vi "EOL Set Power Supply Voltage.vi"(4 "PS Channel Control":i32, 6 "station name":string, 7 "power supply type":T1, 8 "Error Table In":string[][](table), 9 "station idx":i32=4, 10 "Power Supply Voltage":dbl, 11 "Power Supply Comm Port":refnum<visa-resource-name>="COM1") -> (0 "Error Table Out":string[][](array[string]), 2 "Actual Voltage":dbl, 3 "Pass?":bool)   [LabVIEW 2018]
uses:
  05.UserVI's/Lambda Power/power supply types.ctl
  Fergus/ZUP_Current/Def Ctrl/CMD Type.ctl
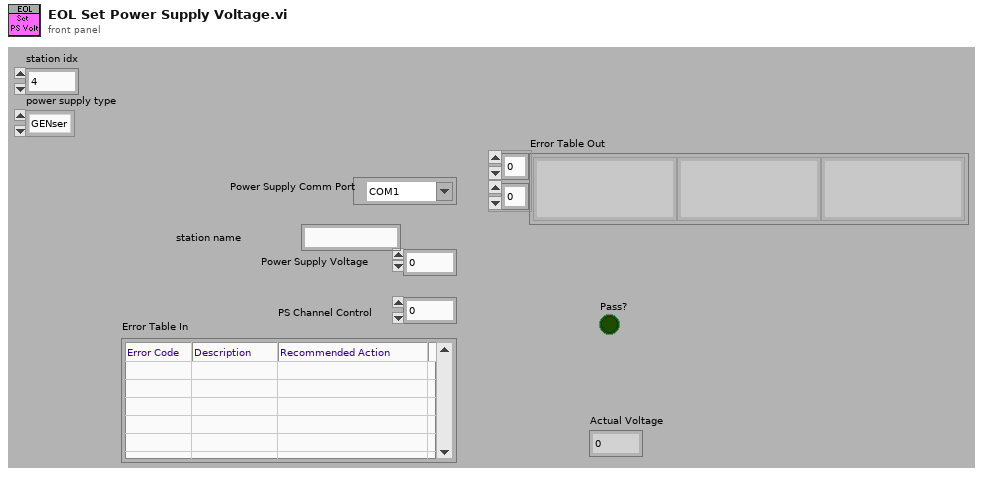
[diagram p1: front panel]
types:
  T1 = typedef "power supply types.ctl" = enum16{"GENser", "ZUPser", "GENeth", "Manual", "ITECH"}
  T2 = cluster{"Power Supply Voltage":dbl, "station name":string, "Max Voltage":dbl, "Min Voltage":dbl, "PS Channel Control":i32, "Power Supply Comm Port":refnum<visa-resource-name>, "Error String":string, "Actual Voltage":dbl, "Start Timer":u32, "Pass?":bool, "station idx":i32, "power supply type":T1}
  T3 = typedef "CMD Type.ctl" = enum16{"Default", "SetADR", "SetRMT", "SetVOL", "SetCUR", "SetOUT", "CheckREV", "CheckRMT", "CheckVOL", "CkeckCUR", "CheckOUT"}
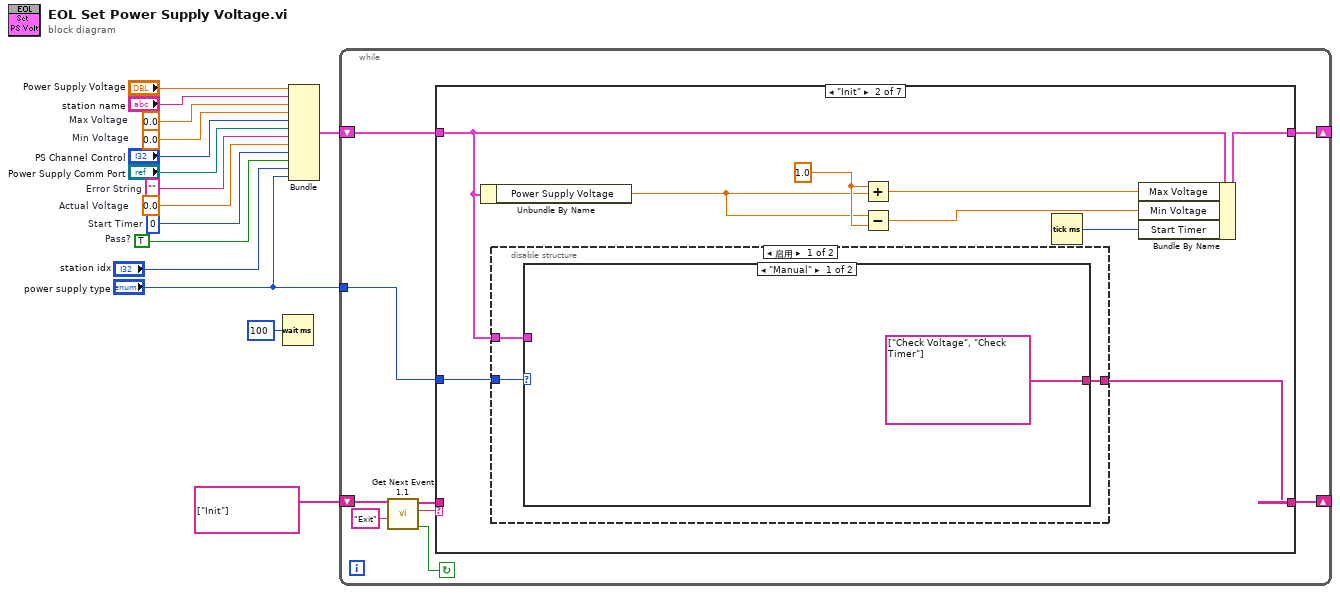
[diagram p0: block diagram]
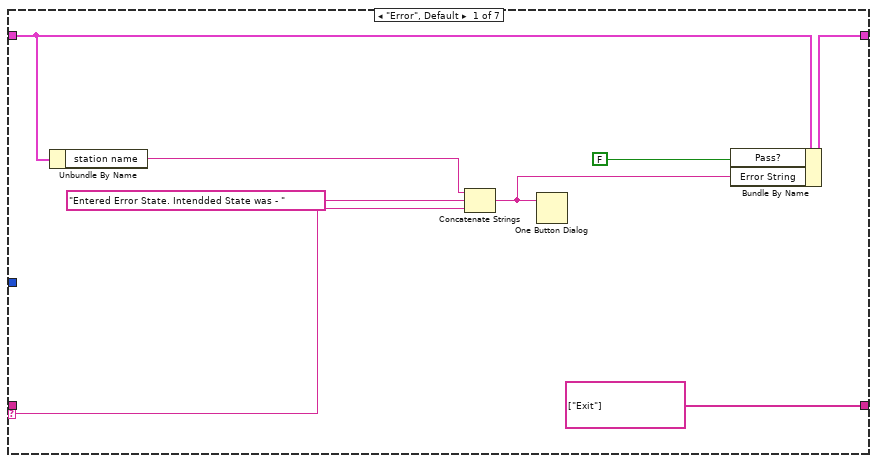
[diagram p2: hidden frame]
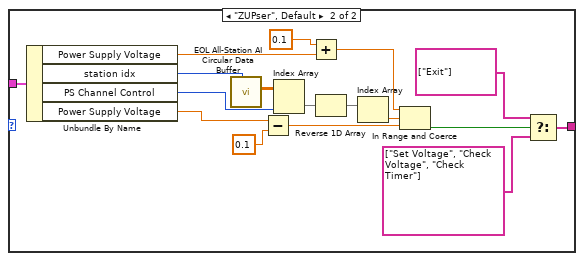
[diagram p3: hidden frame]
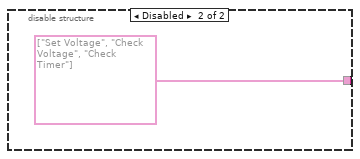
[diagram p4: hidden frame]
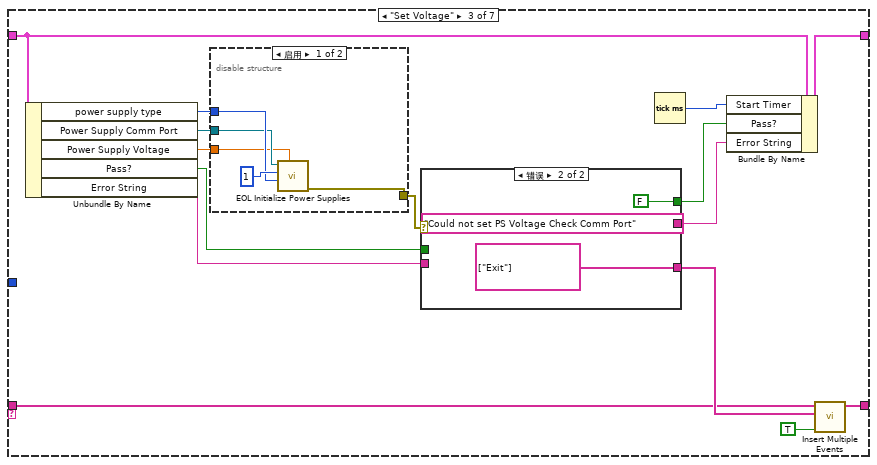
[diagram p5: hidden frame]
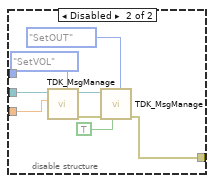
[diagram p6: hidden frame]
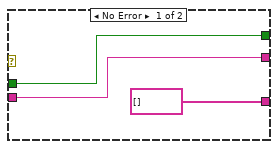
[diagram p7: hidden frame]
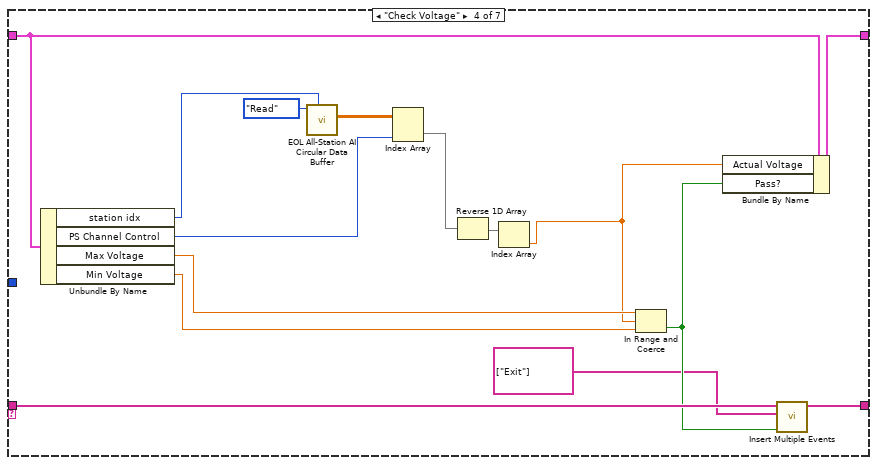
[diagram p8: hidden frame]
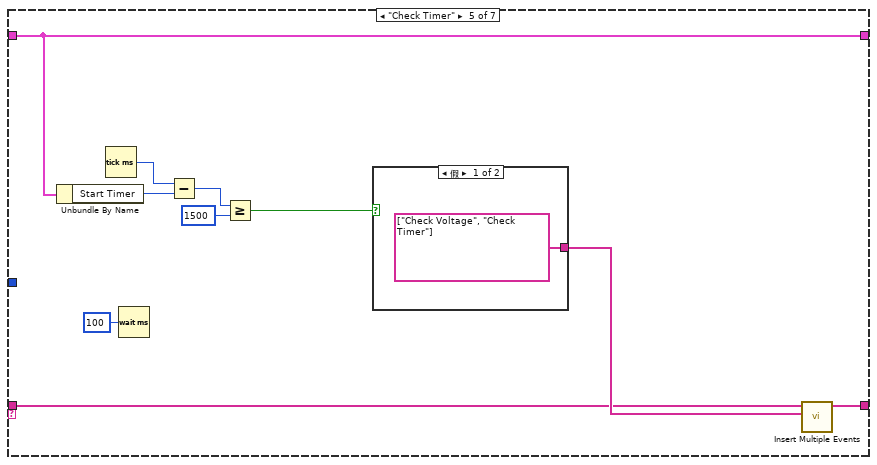
[diagram p9: hidden frame]
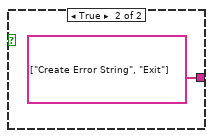
[diagram p10: hidden frame]
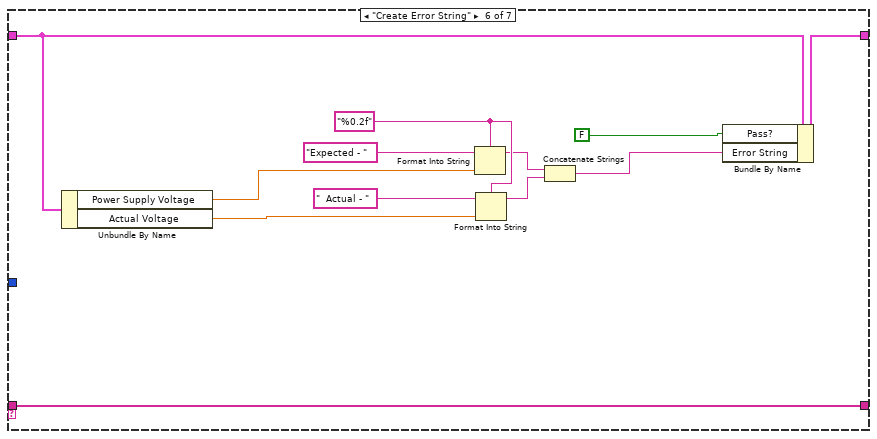
[diagram p11: hidden frame]
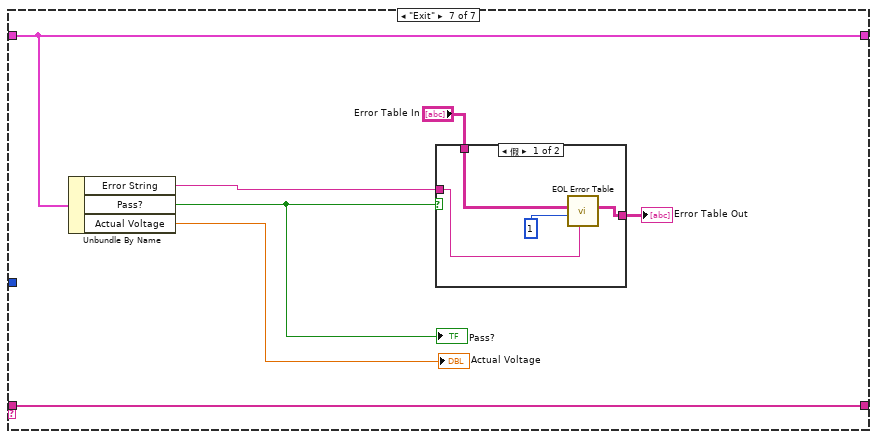
[diagram p12: hidden frame]
diagram:
  w4 = TRUE  # Pass?
  w5 = u32 0  # Start Timer
  w6 = 0.0  # Actual Voltage
  w7 = ""  # Error String
  w11 = 0.0  # Max Voltage
  w10 = 0.0  # Min Voltage
  n1 = Wait (ms)(milliseconds to wait=u32 100) -> ()  [unwired: 1 out]
  n2 = Bundle("Power Supply Voltage"="Power Supply Voltage", "station name"="station name", "Max Voltage"=w11, "Min Voltage"=w10, "PS Channel Control"="PS Channel Control", "Power Supply Comm Port"="Power Supply Comm Port", "Error String"=w7, "Actual Voltage"=w6, "Start Timer"=w5, "Pass?"=w4, "station idx"="station idx", "power supply type"="power supply type") -> (w12:T2)  [unwired: 1 in]
  n3 = while {
    shift-right: [w20] -> _
    shift-left: string[] ["Init"] ("event queue out") -> [w19]
    shift-right: [w17] -> _
    shift-left: w12 -> [w18]
    tunnel: "power supply type" -> [w16]
    stop <- w24 continue-if-true
    n4 = call "Get Next Event 1.1.vi"("Exit Event"="Exit", "event queue in"=w19) -> ("Condition (Exit:F)"=w24:bool, "next event"=w22:string, "event queue out"=w21:string[])  [unwired: 6 in, 1 out]
    n5 = case shown="\"Init\"" w22 {
      selector: w22 -> [w31 _ _ _ _ _ _]
      tunnel: w21 -> [_ _ w76 w106 w115 w136 w143]
      tunnel: [string[] ["Exit"] ("event queue out") w34 w78 w107 w116 w136 w143] -> w20
      tunnel: w18 -> [w29 w35 w74 w109 w114 w135 w140]
      tunnel: [w28 w39 w73 w108 w114 w134 w140] -> w17
      tunnel: w16 -> [_ w33 _ _ _ _ _]
      frame "Error", Default {
        n6 = Unbundle By Name(w29) -> ("station name"=w25:string)
        n7 = Concatenate Strings(w25, "Entered Error State. Intendded State was - " ("string"), w31) -> (w26:string)
        n8 = One Button Dialog(message=w26) -> ()  [unwired: 1 in, 1 out]
        n9 = Bundle By Name(cluster=w29, "Pass?"=FALSE, "Error String"=w26) -> (w28:T2)
      }
      frame "Init" {
        w41 = 1.0 ("x")
        n10 = Unbundle By Name(w35) -> ("Power Supply Voltage"=w40:dbl)
        n11 = disable-structure shown="启用" {
          disable-tunnel: w35 -> [w44 _]
          disable-tunnel: [w43 string[] ["Set Voltage", "Check Voltage", "Check Timer"] ("event queue out")] -> w34
          disable-tunnel: w33 -> [w42 _]
          frame Enabled {
            n12 = case shown="\"Manual\"" w42 {
              tunnel: w44 -> [_ w50]
              tunnel: [string[] ["Check Voltage", "Check Timer"] ("event queue out") w46] -> w43
              frame "Manual" {
              }
              frame "ZUPser", Default {
                n13 = Unbundle By Name(w50) -> ("Power Supply Voltage"=w57:dbl, "station idx"=w54:i32, "PS Channel Control"=w55:i32, "Power Supply Voltage"=w60:dbl)
                n14 = call "EOL All-Station AI Circular Data Buffer.vi"("station idx"=w54) -> ("Data Read (Samp-Ro, Ch-Col)"=w52:sgl[][])  [unwired: 10 in]
                n15 = Subtract(x=w60, y=0.1) -> (x-y=w62:dbl)
                n16 = Index Array(array=w52, index (col)=w55) -> (element=w53:sgl[])  [unwired: 1 in]
                n17 = Add(x=0.1 ("y"), y=w57) -> (x+y=w59:dbl)
                n18 = Reverse 1D Array(array=w53) -> (reversed array=w51:sgl[])
                n19 = Index Array(array=w51) -> (element=w56:sgl)  [unwired: 1 in]
                n20 = In Range and Coerce(upper limit=w59, x=w56, lower limit=w62) -> (In Range?=w49:bool)  [unwired: 1 out]
                n21 = Select(t=string[] ["Exit"] ("event queue out"), s=w49, f=string[] ["Set Voltage", "Check Voltage", "Check Timer"] ("event queue out")) -> (s? t:f=w46:string[])
              }
            }
          }
          frame Disabled {
          }
        }
        n22 = Add(x=w41, y=w40) -> (x+y=w38:dbl)
        n23 = Subtract(x=w40, y=w41) -> (x-y=w37:dbl)
        n24 = Tick Count (ms)() -> (millisecond timer value=w36:u32)
        n25 = Bundle By Name(cluster=w35, "Max Voltage"=w38, "Min Voltage"=w37, "Start Timer"=w36) -> (w39:T2)
      }
      frame "Set Voltage" {
        n26 = Unbundle By Name(w74) -> ("power supply type"=w67:T1, "Power Supply Comm Port"=w66:refnum<visa-resource-name>, "Power Supply Voltage"=w65:dbl, "Pass?"=w69:bool, "Error String"=w71:string)
        n27 = disable-structure shown="启用" {
          disable-tunnel: w67 -> [w82 _]
          disable-tunnel: w66 -> [w81 w90]
          disable-tunnel: w65 -> [w80 w91]
          disable-tunnel: [w79 w84] -> w64
          frame Enabled {
            n28 = call "EOL Initialize Power Supplies.vi"("Volt Limit"=w80, "power supply model"=w82, "No. of Power Supplies"=1, "VISA resource name"=w81) -> ("error out"=w79:errorcluster)  [unwired: 7 in]
          }
          frame Disabled {
            n29 = call "TDK_MsgManage.vi"("CMD Type"=CMD_Type."SetVOL", "Voltage"=w91, "VISA resource name"=w90) -> ("error out"=w88:errorcluster, "VISA resource name"=w87:refnum<visa-resource-name>)  [unwired: 5 in, 2 out]
            n30 = call "TDK_MsgManage.vi"("CMD Type"=CMD_Type."SetOUT", "OUT?"=TRUE, "error in (no error)"=w88, "VISA resource name"=w87) -> ("error out"=w84:errorcluster)  [unwired: 4 in, 3 out]
          }
        }
        n31 = case shown="错误" w64 {
          tunnel: [string[] [] ("event queue out") string[] ["Exit"] ("event queue out")] -> w77
          tunnel: [w93 "Could not set PS Voltage Check Comm Port"] -> w72
          tunnel: w71 -> [w93 _]
          tunnel: w69 -> [w92 _]
          tunnel: [w92 FALSE ("Pass?")] -> w68
          frame No Error {
          }
          frame Error {
          }
        }
        n32 = Tick Count (ms)() -> (millisecond timer value=w70:u32)
        n33 = Bundle By Name(cluster=w74, "Start Timer"=w70, "Pass?"=w68, "Error String"=w72) -> (w73:T2)
        n34 = call "Insert Multiple Events.vi"("Insert all? (T)"=TRUE, "Events to Insert"=w77, "Event queue in"=w76) -> ("Event queue out"=w78:string[])  [unwired: 4 in]
      }
      frame "Check Voltage" {
        n35 = Unbundle By Name(w109) -> ("station idx"=w100:i32, "PS Channel Control"=w99:i32, "Max Voltage"=w111:dbl, "Min Voltage"=w110:dbl)
        n36 = call "EOL All-Station AI Circular Data Buffer.vi"("station idx"=w100, "Mode"=enum16{"Initialize", "Read", "Write"}."Read") -> ("Data Read (Samp-Ro, Ch-Col)"=w102:sgl[][])  [unwired: 9 in]
        n37 = Index Array(array=w102, index (col)=w99) -> (element=w101:sgl[])  [unwired: 1 in]
        n38 = Reverse 1D Array(array=w101) -> (reversed array=w112:sgl[])
        n39 = Index Array(array=w112) -> (element=w98:sgl)  [unwired: 1 in]
        n40 = In Range and Coerce(upper limit=w111, x=w98, lower limit=w110) -> (In Range?=w105:bool)  [unwired: 1 out]
        n41 = Bundle By Name(cluster=w109, "Actual Voltage"=w98, "Pass?"=w105) -> (w108:T2)
        n42 = call "Insert Multiple Events.vi"("Insert all? (T)"=w105, "Events to Insert"=string[] ["Exit"] ("event queue out"), "Event queue in"=w106) -> ("Event queue out"=w107:string[])  [unwired: 4 in]
      }
      frame "Check Timer" {
        n43 = Unbundle By Name(w114) -> ("Start Timer"=w121:u32)
        n44 = Tick Count (ms)() -> (millisecond timer value=w122:u32)
        n45 = Wait (ms)(milliseconds to wait=u32 100) -> ()  [unwired: 1 out]
        n46 = Subtract(x=w122, y=w121) -> (x-y=w120:u32)
        n47 = Greater Or Equal?(x=w120, y=u32 1500) -> (x >= y?=w118:bool)
        n48 = case shown="假" w118 {
          tunnel: [string[] ["Check Voltage", "Check Timer"] ("event queue out") string[] ["Create Error String", "Exit"] ("event queue out")] -> w117
          frame False {
          }
          frame True {
          }
        }
        n49 = call "Insert Multiple Events.vi"("Events to Insert"=w117, "Event queue in"=w115) -> ("Event queue out"=w116:string[])  [unwired: 5 in]
      }
      frame "Create Error String" {
        w132 = "%0.2f" ("format string")
        n50 = Unbundle By Name(w135) -> ("Power Supply Voltage"=w127:dbl, "Actual Voltage"=w126:dbl)
        n51 = Format Into String(format string=w132, initial string="Expected - ", w127) -> (resulting string=w130:string)  [unwired: 1 in, 1 out]
        n52 = Format Into String(format string=w132, initial string="  Actual - ", w126) -> (resulting string=w131:string)  [unwired: 1 in, 1 out]
        n53 = Concatenate Strings(w130, w131) -> (w125:string)
        n54 = Bundle By Name(cluster=w135, "Pass?"=FALSE, "Error String"=w125) -> (w134:T2)
      }
      frame "Exit" {
        n55 = Unbundle By Name(w140) -> ("Error String"=w138:string, "Pass?"=w139:bool, "Actual Voltage"=→"Actual Voltage":dbl)
        "Pass?" <- w139
        n56 = case shown="假" w139 {
          tunnel: "Error Table In" -> [w147 w148]
          tunnel: [w144 w148] -> w142
          tunnel: w138 -> [w146 _]
          frame False {
            n57 = call "EOL Error Table.vi"("Error Description"=w146, "Error No."=u16 1, "Error Table In"=w147) -> ("Error Table Out"=w144:string[][])  [unwired: 7 in, 1 out]
          }
          frame True {
          }
        }
        "Error Table Out" <- w142
      }
    }
  }
